vi "DiagServiceLayer.vi"(0 "path":path, 1 "ADiagModuleIndex":i32, 2 "Diag传输层参数":T1={"FilledByte"=0, "STMin"=10, "BlockSize"=10, "FCDelay"=10, "MaxLength"=4095} {"FilledByte" format="%.0x"}, 3 "错误输入":errorcluster caption="错误输入（无错误）") -> (7 "path out":path, 8 "returns":i32[](array[numeric]), 10 "错误输出":errorcluster)   [LabVIEW 2014]
panel:
  # "S"
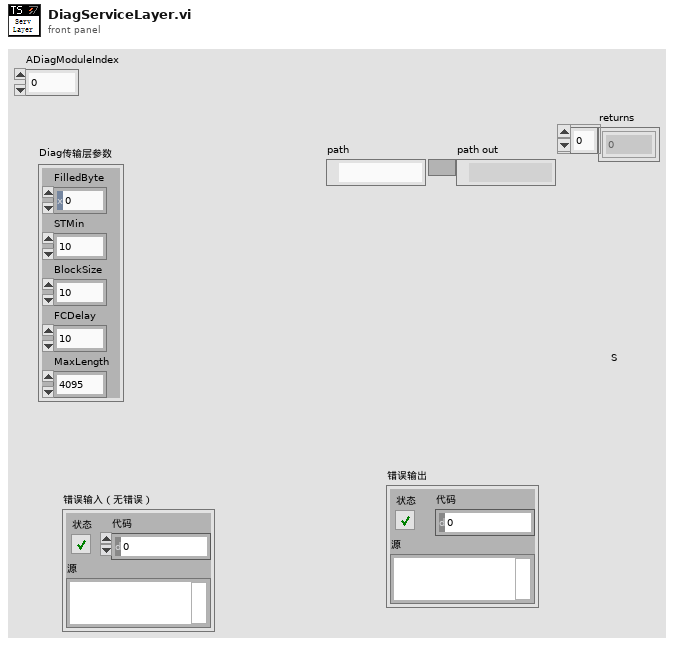
[diagram p1: front panel]
types:
  T1 = cluster{"FilledByte":u8, "STMin":i32, "BlockSize":i32, "FCDelay":i32, "MaxLength":i32}
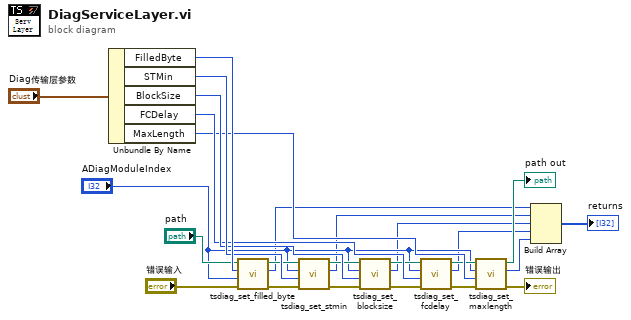
[diagram p0: block diagram]
diagram:
  n1 = Unbundle By Name("Diag传输层参数") -> ("FilledByte"=w24:u8, "STMin"=w23:i32, "BlockSize"=w22:i32, "FCDelay"=w21:i32, "MaxLength"=w20:i32)
  n2 = call "tsdiag_set_filled_byte.vi"("错误输入（无错误）"="错误输入", "pDiagModuleIndex"="ADiagModuleIndex", "AFilledByte"=w24, "path"="path") -> ("错误输出"=w15:errorcluster, "Return Type"=w6:i32, "path output"=w17:path)  [unwired: 5 in]
  n3 = call "tsdiag_set_stmin.vi"("error in (no error)"=w15, "AST"=w23, "ADiagModuleIndex"="ADiagModuleIndex", "路径输入"=w17) -> ("error out"=w13:errorcluster, "retirn"=w5:i32, "路径输出"=w14:path)  [unwired: 5 in]
  n4 = call "tsdiag_set_blocksize.vi"("error in (no error)"=w13, "ABlockSize"=w22, "ADiagModuleIndex"="ADiagModuleIndex", "路径输入"=w14) -> ("error out"=w11:errorcluster, "return"=w4:i32, "路径输出"=w12:path)  [unwired: 5 in]
  n5 = call "tsdiag_set_fcdelay.vi"("error in (no error)"=w11, "AFCDelay"=w21, "ADiagModuleIndex"="ADiagModuleIndex", "路径输入"=w12) -> ("error out"=w10:errorcluster, "return"=w3:i32, "路径输出"=w9:path)  [unwired: 5 in]
  n6 = call "tsdiag_set_maxlength.vi"("error in (no error)"=w10, "Maxlength"=w20, "ADiagModuleIndex"="ADiagModuleIndex", "路径输入"=w9) -> ("error out"=→"错误输出":errorcluster, "return"=w2:i32, "路径输出"=→"path out":path)  [unwired: 5 in]
  n7 = Build Array(w6, w5, w4, w3, w2) -> (→"returns":i32[])
